vi "dvr_fgv_write.vi"(8 "error in (no error)":errorcluster, 11 "Boolean":bool) -> (0 "error out":errorcluster)   [LabVIEW 2020]
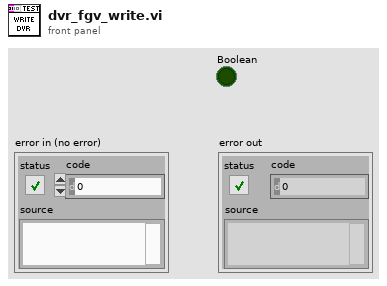
[diagram p1: front panel]
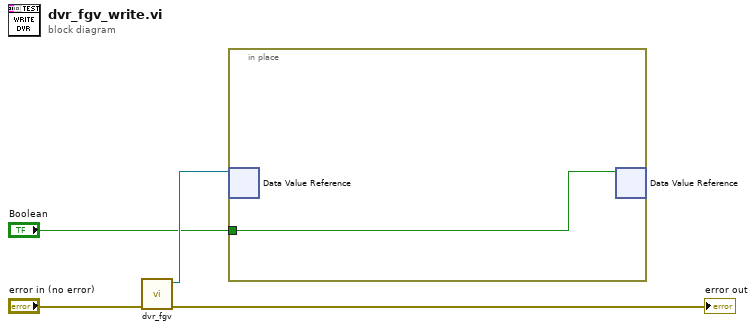
[diagram p0: block diagram]
diagram:
  n1 = call "dvr_fgv.vi"("error in (no error)"="error in (no error)") -> ("error out"=→"error out":errorcluster, "data value reference"=w2:refnum<data-value>)  [unwired: 9 in]
  n2 = in-place {
    in-place-border: "Boolean" -> [w5]
    n3 = in-place-dvr #1(w2) -> ()  [unwired: 2 out]
    n4 = in-place-dvr #1(w5) -> ()  [unwired: 2 out]
  }
